vi "Client List.vi"(8 "error in (no error)":errorcluster, 11 "TCPMessageAPI in":refnum<class "TCPMessageAPI.lvclass">) -> (0 "error out":errorcluster, 2 "Client List":T1, 3 "TCPMessageAPI out":refnum<class "TCPMessageAPI.lvclass">)   [LabVIEW 2020, in "Vecto.lvlib" / "TCPMessageAPI.lvclass"]
uses:
  TCPMessageAPI.lvclass
  lv-volatus/messages/TcpClientList/Data.ctl
  lv-volatus/messages/TcpClientInfo/Data.ctl
  TCPMessageAPI.lvclass/TCPMessageAPI.ctl
  lv-volatus/messages/TcpClientInfo/TcpClientInfo.lvlib
  lv-volatus/messages/TcpClientList/TcpClientList.lvlib
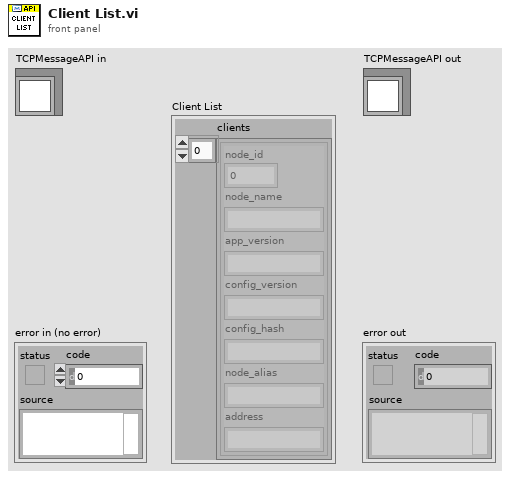
[diagram p1: front panel]
types:
  T1 = typedef "TcpClientList.lvlib/Data.ctl" = cluster{"clients":T2[]}
  T2 = typedef "TcpClientInfo.lvlib/Data.ctl" = cluster{"node_id":u32, "node_name":string, "app_version":string, "config_version":string, "config_hash":string, "node_alias":string, "address":string}
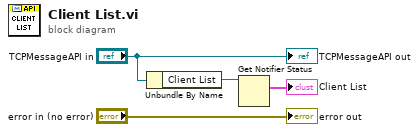
[diagram p0: block diagram]
diagram:
  n1 = Unbundle By Name("TCPMessageAPI in") -> ("Client List"=w2:refnum<notifier>)
  n2 = Get Notifier Status(notifier=w2) -> (current notification=→"Client List":T1)  [unwired: 1 in, 4 out]
  "error out" <- "error in (no error)"
  "TCPMessageAPI out" <- "TCPMessageAPI in"
